vi "DAQ.vi"() -> ()   [LabVIEW 2018]
uses:
  55be89dd-8425-478b-abe4-e99fbfe30e24.vi
  <extravilib>/ChannelInstances/Messenger-bool/Write With Abort.vi
  <extravilib>/ChannelInstances/Messenger-bool/Read With Abort.vi
  <resource>/Channels/Messenger/Write With Abort.vi
  <resource>/Channels/Messenger/Read With Abort.vi
  <vilib>/ChannelSupport/Channel Message/Read ID.vi
  <extravilib>/ChannelInstances/Messenger-bool/Wrapper.lvclass
  C:/Program Files (x86)/National Instruments/LabVIEW 2018/vi.lib/ChannelSupport/Channel Message/Channel Message.lvclass
  <extravilib>/ChannelInstances/Messenger-bool/Instantiate.vi
  <resource>/Channels/Messenger/Endpoint.vi
  <extravilib>/ChannelInstances/Messenger-bool/Unwrap.vi
  <vilib>/Utility/inputDevices.llb/keyboardAcquire.vi
  <extravilib>/ChannelInstances/Messenger-bool/Wrap.vi
  PostgreSQL2LabVIEW/libpqlv/libpqlv.lvlib
  <vilib>/Utility/error.llb/DialogType.ctl
  <extravilib>/ChannelInstances/Messenger-bool.lvlib
panel:
  out "Chamber Temperature":dbl format="%#.1f °C"
  out "Chamber Pressure":dbl format="%#.1f psi"
  in  "CV-006\nAir Supply Valve":bool
  out "Pneumatic\nAir Pressure":dbl caption="Lox Tank Level" format="%#.1f psi"
  in  "CV-001\nFuel Vent Valve":bool
  out "Fuel Tank Pressure":dbl caption="Lox Tank Level" format="%#.1f psi"
  out "Thrust":dbl format="%#.0f N"
  out "Fuel Tank Level":dbl caption="Lox Tank Level" format="%#.1f kg"
  out "Fuel Tank Temperature":dbl format="%#.1f  °C"
  out "Lox Tank Level":dbl format="%#.1f  kg"
  out "LOX Tank Temperature":dbl format="%#.1f °C"
  in  "Start / Abort Button":bool
  out "data out":string
  out "Database Time":string
  out "Timer":string
  in  "stop":bool
  out "Fuel Feed Pressure":dbl format="%#.1f psi"
  out "LOX Feed Pressure":dbl format="%#.1f psi"
  out "Helium Pressure":dbl format="%#.0f psi"
  out "LOX Tank Pressure":dbl format="%#.1f psi"
  in  "CV-005\nLOX Fill Valve":bool
  in  "CV-003\nMain LOX Valve":bool
  in  "CV-002\nLOX Vent Valve":bool
  in  "CV-000\nHelium Valve":bool
  in  "CV-004\nMain Fuel Valve":bool
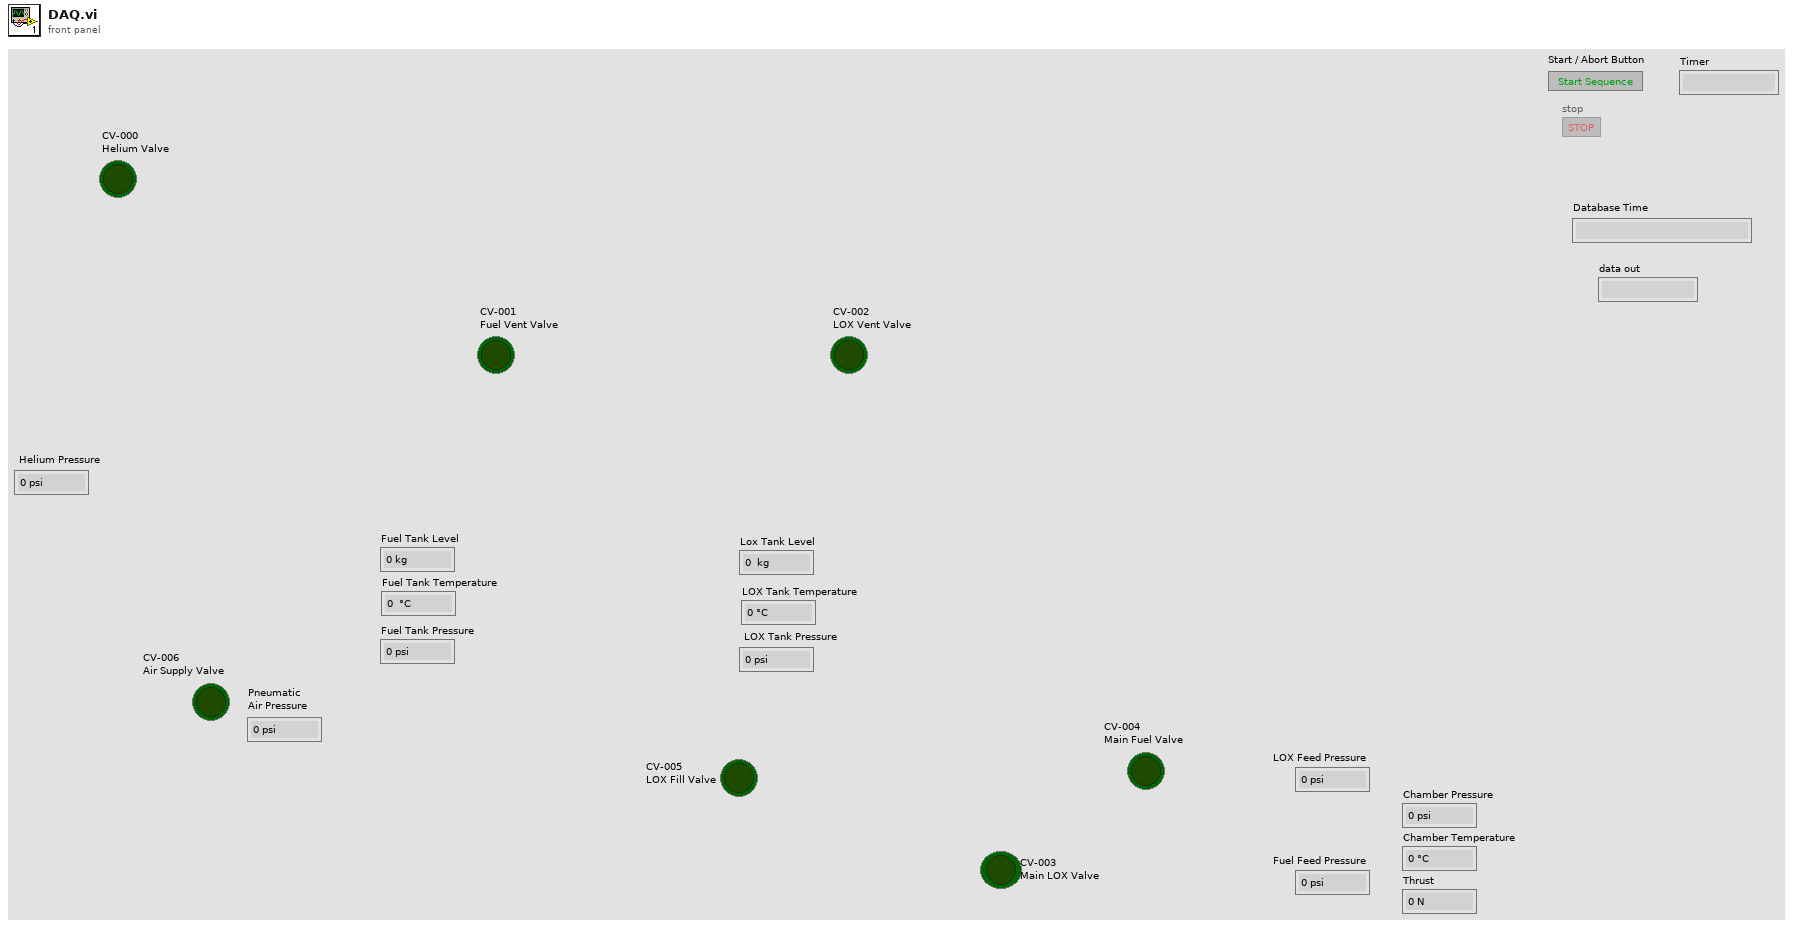
[diagram p1: front panel]
types:
  T1 = enum8{"Enabled", "Disabled", "Disabled and Grayed Out"}
  T2 = enum16{"0", "1", "2", "3", "4", "5", "6", "7", "8", "9", "A", "B", "C", "D", "E", "F", "G", "H", "I", "J", "K", "L", "M", "N", "O", "P", "Q", "R", "S", "T", "U", "V", "W", "X", "Y", "Z", "F1", "F2", "F3", "F4", "F5", "F6", "F7", "F8", "F9", "F10", "F11", "F12", "F13", "F14", "F15", "ADD", "BACK", "BACKSLASH", "CAPITAL", "COMMA", "DECIMAL", "DELETE", "DIVIDE", "DOWN", "END", "EQUALS", "ESCAPE", "GRAVE (`)", "HOME", "INSERT", "LBRACKET", "LCONTROL", "LEFT", "L ALT", "LSHIFT", "LWIN", "MINUS", "MULTIPLY", "NEXT", "NUMLOCK", "NUMPAD_0", "NUMPAD_1", "NUMPAD_2", "NUMPAD_3", "NUMPAD_4", "NUMPAD_5", "NUMPAD_6", "NUMPAD_7", "NUMPAD_8", "NUMPAD_9", "PAUSE", "PERIOD", "PRIOR (PG UP)", "RBRACKET", "RCONTROL", "RETURN", "RIGHT", "R ALT", "RSHIFT", "RWIN", "SCROLL", "SEMICOLON", "SLASH", "SPACE", "SUBTRACT", "TAB", "UP", "ENTER (num pad)", "' (quote)"}
  T3 = enum16{"0", "1", "2", "3", "4", "5", "6", "7", "8", "9", "A", "B", "C", "D", "E", "F", "G", "H", "I", "J", "K", "L", "M", "N", "O", "P", "Q", "R", "S", "T", "U", "V", "W", "X", "Y", "Z", "F1", "F2", "F3", "F4", "F5", "F6", "F7", "F8", "F9", "F10", "F11", "F12", "F13", "F14", "F15", "ADD", "BACK", "BACKSLASH", "CAPITAL", "COMMA", "DECIMAL", "DELETE", "DIVIDE", "DOWN", "END", "EQUALS", "ESCAPE", "GRAVE (`)", "HOME", "INSERT", "LBRACKET", "LCONTROL", "LEFT", "L ALT", "LSHIFT", "LWIN", "MINUS", "MULTIPLY", "NEXT", "NUMLOCK", "NUMPAD_0", "NUMPAD_1", "NUMPAD_2", "NUMPAD_3", "NUMPAD_4", "NUMPAD_5", "NUMPAD_6", "NUMPAD_7", "NUMPAD_8", "NUMPAD_9", "PAUSE", "PERIOD", "PRIOR (PG UP)", "RBRACKET", "RCONTROL", "RETURN", "RIGHT", "R ALT", "RSHIFT", "RWIN", "SCROLL", "SEMICOLON", "SLASH", "SPACE", "SUBTRACT", "TAB", "UP", "ENTER (num pad)", "' (quote)"}[]
  T4 = typedef "Messenger-bool.lvlib/))Channel.ctl" = refnum<queue>
  T5 = enum16{"Standard", "Buffered", "CRLF", "Immediate"}
  T6 = typedef "DialogType.ctl" = u16
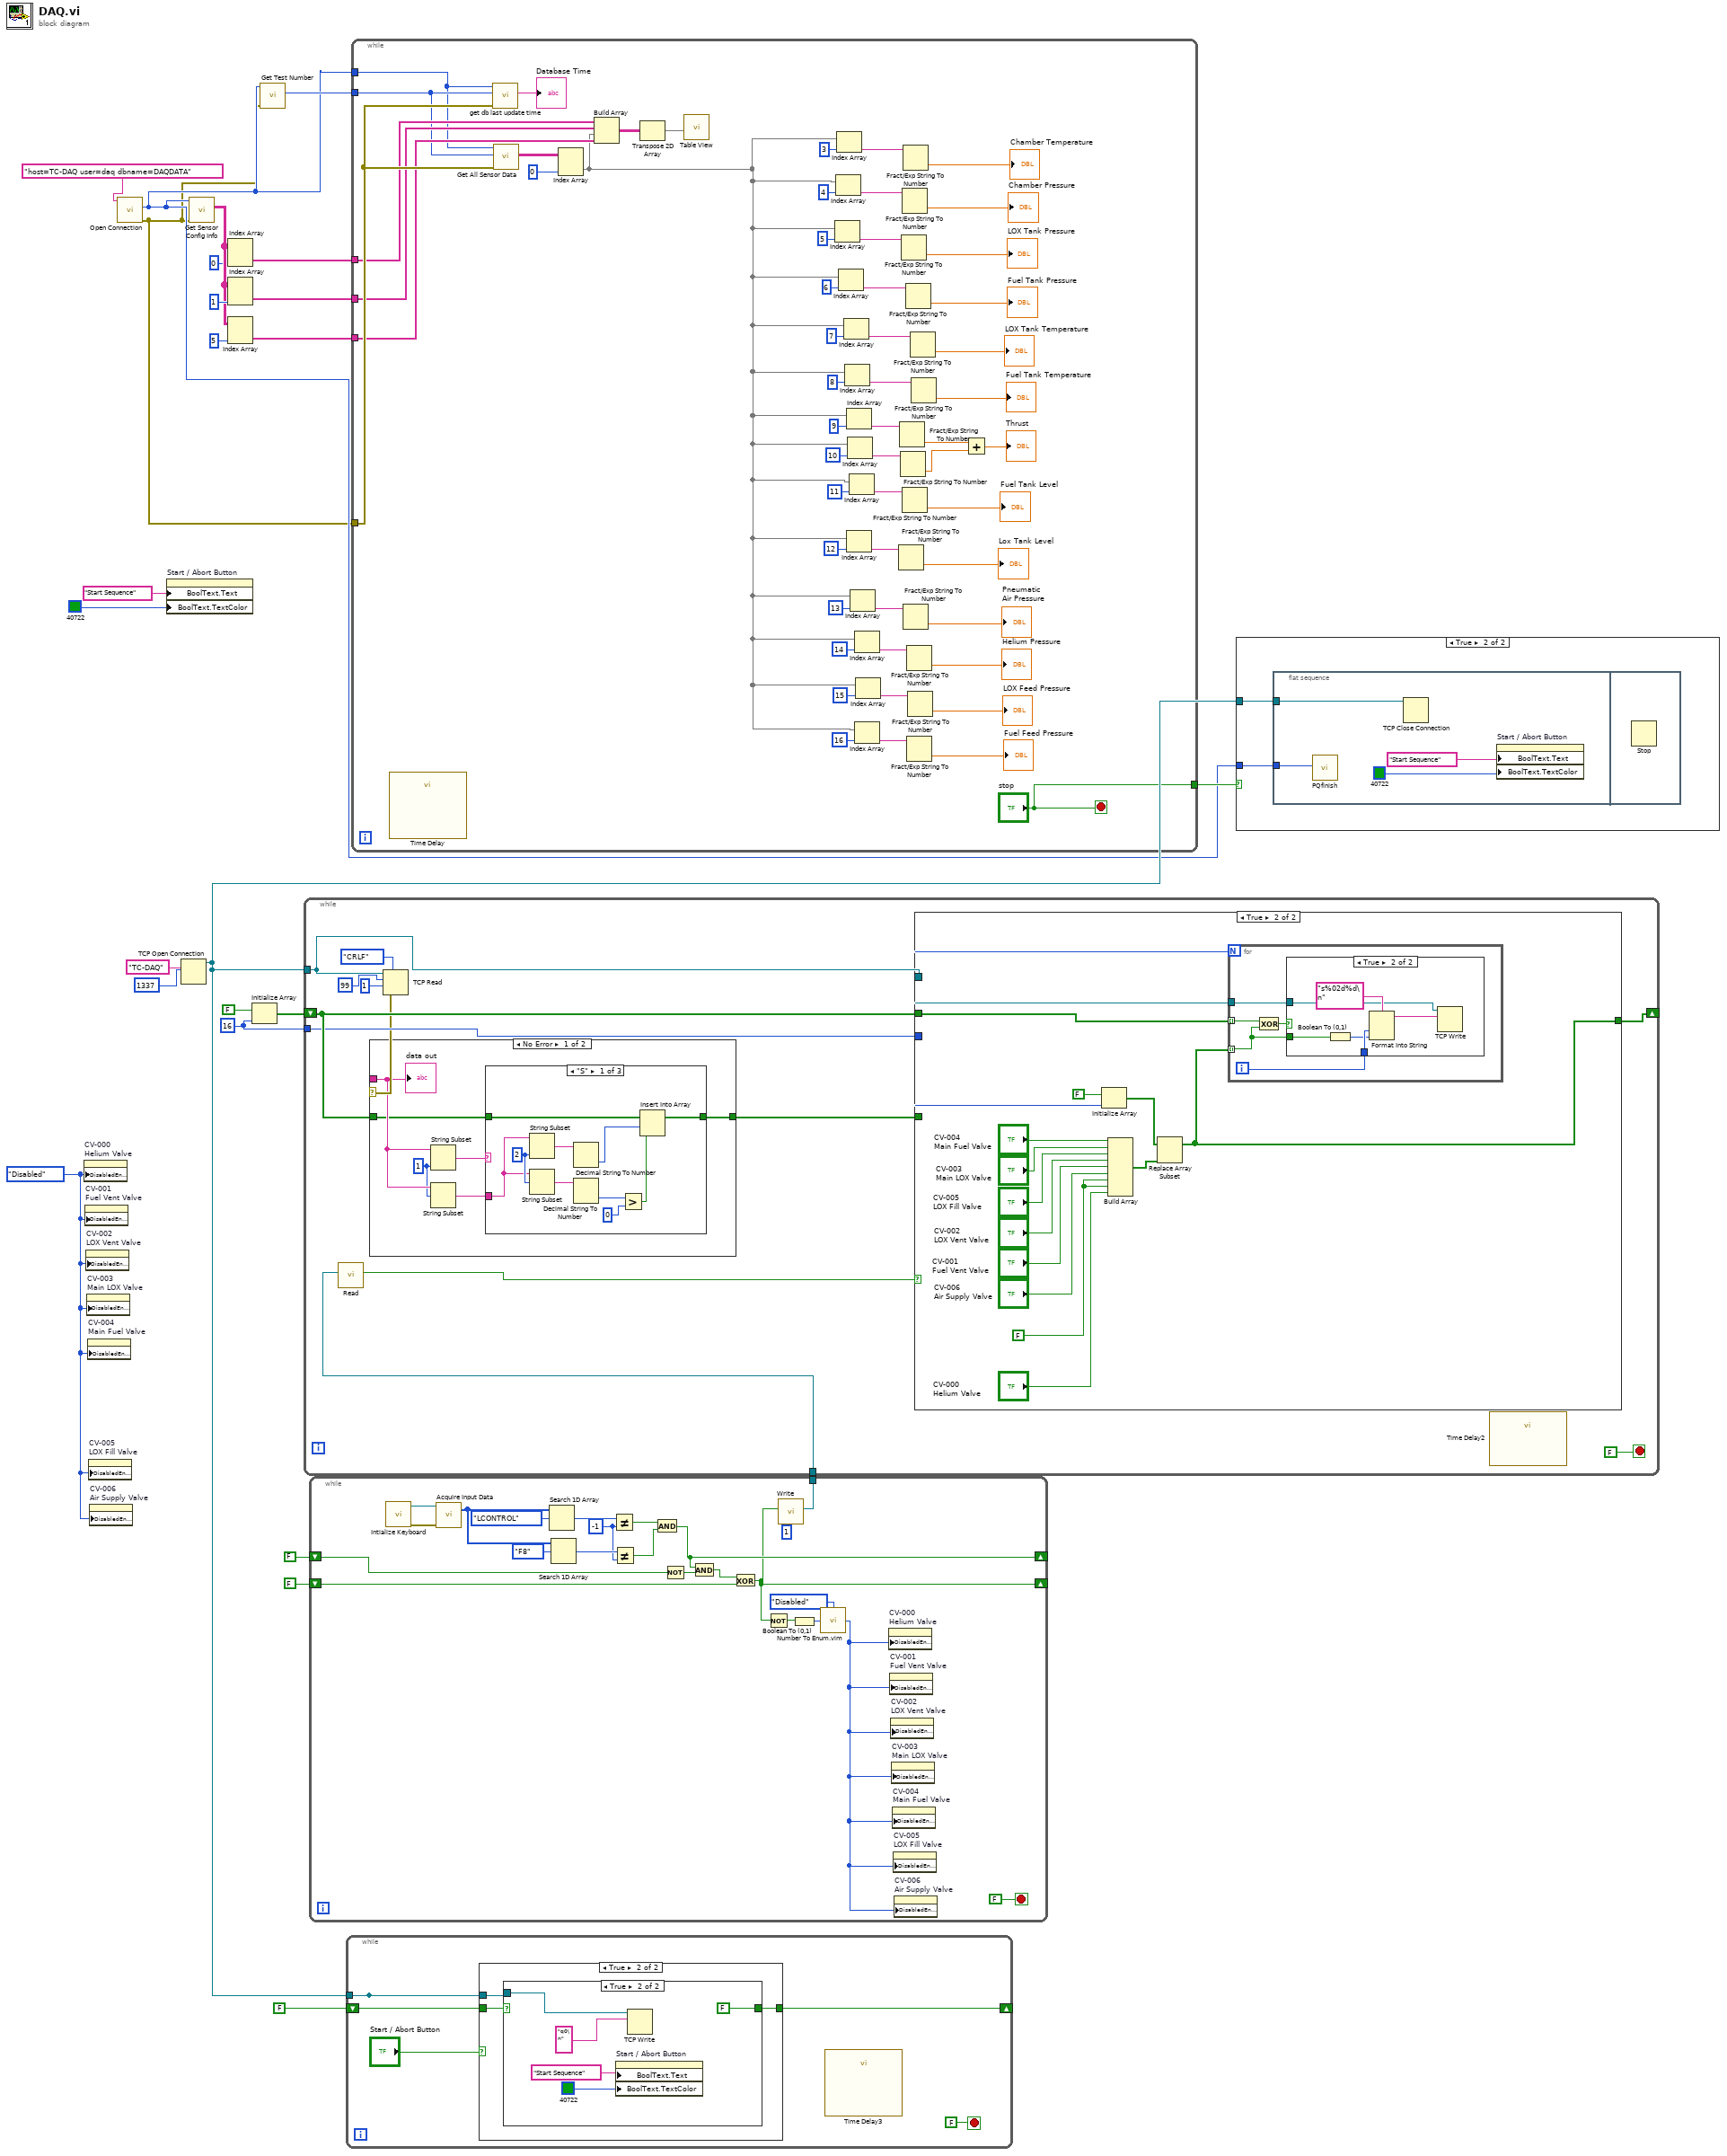
[diagram p0: block diagram]
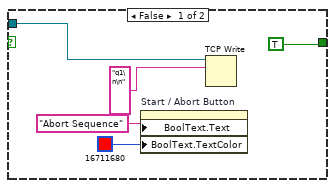
[diagram p3: hidden frame]
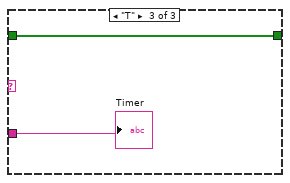
[diagram p5: hidden frame]
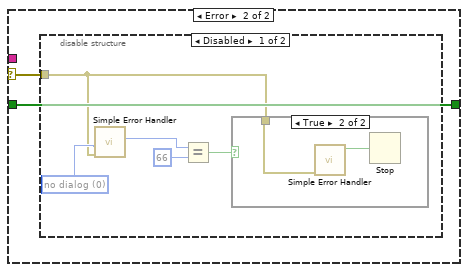
[diagram p6: hidden frame]
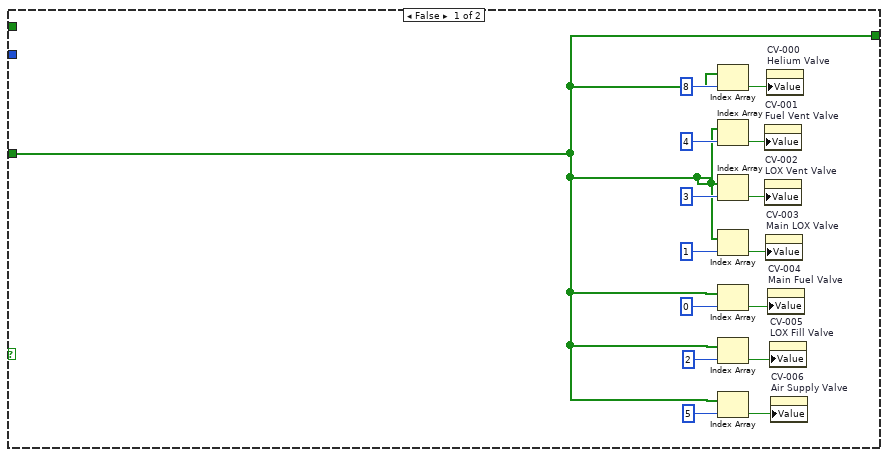
[diagram p9: hidden frame]
diagram:
  w7 = T1."Disabled" ("Disabled")
  w3 = 16 ("dimension size")
  n1 = property on="CV-000\nHelium Valve" class="Bool (strict)"("DisabledEnum"=w7) -> ()  [unwired: 2 in, 2 out]
  n2 = property on="CV-001\nFuel Vent Valve" class="Bool (strict)"("DisabledEnum"=w7) -> ()  [unwired: 2 in, 2 out]
  n3 = property on="CV-002\nLOX Vent Valve" class="Bool (strict)"("DisabledEnum"=w7) -> ()  [unwired: 2 in, 2 out]
  n4 = property on="CV-003\nMain LOX Valve" class="Bool (strict)"("DisabledEnum"=w7) -> ()  [unwired: 2 in, 2 out]
  n5 = property on="CV-004\nMain Fuel Valve" class="Bool (strict)"("DisabledEnum"=w7) -> ()  [unwired: 2 in, 2 out]
  n6 = property on="CV-005\nLOX Fill Valve" class="Bool (strict)"("DisabledEnum"=w7) -> ()  [unwired: 2 in, 2 out]
  n7 = property on="CV-006\nAir Supply Valve" class="Bool (strict)"("DisabledEnum"=w7) -> ()  [unwired: 2 in, 2 out]
  n8 = call "Open Connection.vi"("conninfo"="host=TC-DAQ user=daq dbname=DAQDATA") -> ("error out"=w1:errorcluster, "conn"=w2:u32)  [unwired: 8 in, 1 out]
  n9 = property on="Start / Abort Button" class="Bool"("BoolText.Text"="Start Sequence" ("Boolean Text.Text"), "BoolText.TextColor"=u32 40722) -> ()  [unwired: 2 in, 2 out]
  n10 = TCP Open Connection(address="TC-DAQ", remote port or service name=u16 1337) -> (connection ID=w17:refnum<k5>)  [unwired: 3 in, 1 out]
  n11 = call "Get Sensor Config Info.vi"("error in"=w1, "conn"=w2) -> ("Data"=w10:string[][])  [unwired: 7 in, 2 out]
  n12 = Index Array(array=w10, index (col)=0 ("disabled index (col)")) -> (element=w8:string[])  [unwired: 1 in]
  n13 = Index Array(array=w10, index (col)=1) -> (element=w13:string[])  [unwired: 1 in]
  n14 = Index Array(array=w10, index (col)=5 ("disabled index (col)")) -> (element=w11:string[])  [unwired: 1 in]
  n15 = Initialize Array(FALSE, w3) -> (w15:bool[])
  n16 = call "Get Test Number.vi"("error in"=w1, "conn"=w2) -> ("test_num"=w24:i32)  [unwired: 7 in, 2 out]
  n17 = while {
    shift-right: [w37] -> _
    shift-left: FALSE -> [w35]
    shift-right: [w31] -> _
    shift-left: FALSE -> [w33]
    tunnel: [w27] -> w4
    stop <- FALSE stop-if-true
    w40 = -1 ("y")
    n18 = call <vilib>:"Intialize Keyboard.vi"() -> ("error out"=w46:errorcluster, "device ID"=w48:refnum<k1>)  [unwired: 10 in]
    n19 = call-poly <vilib>:"Acquire Input Data.vi"("device ID"=w48, "error in (no error)"=w46) -> ("keys pressed"=w44:T3)  [unwired: 15 in, 2 out]
    n20 = Search 1D Array(1D array=w44, element=T2."LCONTROL") -> (index of element=w42:i32)  [unwired: 1 in]
    n21 = Search 1D Array(1D array=w44, element=T2."F8") -> (index of element=w41:i32)  [unwired: 1 in]
    n22 = Not Equal?(x=w42, y=w40) -> (x != y?=w39:bool)
    n23 = Not Equal?(x=w41, y=w40) -> (x != y?=w38:bool)
    n24 = And(x=w39, y=w38) -> (x .and. y?=w37:bool)
    n25 = Not(x=w35) -> (.not. x?=w36:bool)
    n26 = And(x=w37, y=w36) -> (x .and. y?=w34:bool)
    n27 = Exclusive Or(1:w33, 2:w34) -> (0:w31:bool)
    n28 = Not(x=w31) -> (.not. x?=w32:bool)
    n29 = call <extravilib>:"Write.vi"("size (unlimited)"=1, "element"=w31) -> ("channel"=w27:T4)  [unwired: 7 in, 2 out]
    n30 = Boolean To (0,1)(Boolean=w32) -> (0, 1=w30:i16)
    n31 = call "Number To Enum.vim"("number"=w30, "enum type"=T1."Disabled" ("Disabled")) -> ("number as enum"=w29:T1)
    n32 = property on="CV-000\nHelium Valve" class="Bool (strict)"("DisabledEnum"=w29) -> ()  [unwired: 2 in, 2 out]
    n33 = property on="CV-001\nFuel Vent Valve" class="Bool (strict)"("DisabledEnum"=w29) -> ()  [unwired: 2 in, 2 out]
    n34 = property on="CV-002\nLOX Vent Valve" class="Bool (strict)"("DisabledEnum"=w29) -> ()  [unwired: 2 in, 2 out]
    n35 = property on="CV-003\nMain LOX Valve" class="Bool (strict)"("DisabledEnum"=w29) -> ()  [unwired: 2 in, 2 out]
    n36 = property on="CV-004\nMain Fuel Valve" class="Bool (strict)"("DisabledEnum"=w29) -> ()  [unwired: 2 in, 2 out]
    n37 = property on="CV-005\nLOX Fill Valve" class="Bool (strict)"("DisabledEnum"=w29) -> ()  [unwired: 2 in, 2 out]
    n38 = property on="CV-006\nAir Supply Valve" class="Bool (strict)"("DisabledEnum"=w29) -> ()  [unwired: 2 in, 2 out]
  }
  n39 = while {
    tunnel: w17 -> [w61]
    shift-right: [w49] -> _
    shift-left: w15 -> [w60]
    tunnel: w4 -> [w58]
    tunnel: w3 -> [w56]
    stop <- FALSE stop-if-true
    n40 = call <extravilib>:"Read.vi"("channel"=w58) -> ("element"=w57:bool)  [unwired: 7 in, 3 out]
    n41 = TCP Read(connection ID=w61, bytes to read=99, 7:T5."CRLF" ("mode (standard)"), 9:1 ("timeout ms (25000)")) -> (data out=w54:string, error out=w55:errorcluster)  [unwired: 1 in, 1 out]
    n42 = case shown="No Error" w55 {
      selector: w55 -> [_ w81]
      tunnel: w54 -> [w66 _]
      tunnel: w60 -> [w63 w82]
      tunnel: [w62 w82] -> w51
      frame No Error {
        w65 = 1 ("length (rest)")
        n43 = String Subset(string=w66, length (rest)=w65) -> (substring=w67:string)  [unwired: 1 in]
        n44 = String Subset(string=w66, offset (0)=w65) -> (substring=w64:string)  [unwired: 1 in]
        n45 = case shown="\"S\"" w67 {
          tunnel: w64 -> [w68 _ w80]
          tunnel: w63 -> [w77 w78 w79]
          tunnel: [w69 w78 w79] -> w62
          frame "S" {
            w74 = 2 ("length (rest)")
            n46 = String Subset(string=w68, length (rest)=w74) -> (substring=w76:string)  [unwired: 1 in]
            n47 = String Subset(string=w68, offset (0)=w74) -> (substring=w73:string)  [unwired: 1 in]
            n48 = Decimal String To Number(string=w76) -> (number=w75:i32)  [unwired: 2 in, 1 out]
            n49 = Decimal String To Number(string=w73) -> (number=w72:i32)  [unwired: 2 in, 1 out]
            n50 = Greater?(x=w72, y=0) -> (0:w70:bool)
            n51 = Insert Into Array(array=w77, index=w75, new element=w70) -> (w69:bool[])
          }
          frame "False", Default {
          }
          frame "T" {
            "Timer" <- w80
          }
        }
        "data out" <- w66
      }
      frame Error {
        n52 = disable-structure shown="Disabled" {
          disable-tunnel: w81 -> [w83 _]
          frame Disabled {
            w85 = T6 0 items=["no dialog", "OK message", "continue or stop message", "OK message + warnings", "continue/stop + warnings"] ("type of dialog (OK msg:1)")
            n53 = call <vilib>:"Simple Error Handler.vi"("type of dialog (OK msg:1)"=w85, "error in (no error)"=w83) -> ("code out"=w84:i32)  [unwired: 3 in, 4 out]
            n54 = Equal?(x=w84, y=66) -> (x = y?=w86:bool)
            n55 = case shown="True" w86 {
              tunnel: w83 -> [_ w89]
              frame False {
              }
              frame True {
                n56 = call <vilib>:"Simple Error Handler.vi"("error in (no error)"=w89) -> ("error?"=w88:bool)  [unwired: 4 in, 4 out]
                n57 = Stop(stop? (T)=w88) -> ()
              }
            }
          }
          frame Enabled {
          }
        }
      }
    }
    n58 = case shown="True" w57 {
      tunnel: w61 -> [_ w113]
      tunnel: w60 -> [_ w114]
      tunnel: [w90 w115] -> w49
      tunnel: w56 -> [_ w116]
      tunnel: w51 -> [w90 _]
      frame False {
        n59 = Index Array(array=w90, index=8) -> (element=w97:bool)
        n60 = Index Array(array=w90, index=4) -> (element=w96:bool)
        n61 = Index Array(array=w90, index=3) -> (element=w98:bool)
        n62 = Index Array(array=w90, index=1) -> (element=w95:bool)
        n63 = Index Array(array=w90, index=0) -> (element=w94:bool)
        n64 = Index Array(array=w90, index=2) -> (element=w93:bool)
        n65 = Index Array(array=w90, index=5) -> (element=w91:bool)
        n66 = property on="CV-001\nFuel Vent Valve" class="Bool (strict)"("Value"=w96) -> ()  [unwired: 2 in, 2 out]
        n67 = property on="CV-002\nLOX Vent Valve" class="Bool (strict)"("Value"=w98) -> ()  [unwired: 2 in, 2 out]
        n68 = property on="CV-003\nMain LOX Valve" class="Bool (strict)"("Value"=w95) -> ()  [unwired: 2 in, 2 out]
        n69 = property on="CV-000\nHelium Valve" class="Bool (strict)"("Value"=w97) -> ()  [unwired: 2 in, 2 out]
        n70 = property on="CV-004\nMain Fuel Valve" class="Bool (strict)"("Value"=w94) -> ()  [unwired: 2 in, 2 out]
        n71 = property on="CV-005\nLOX Fill Valve" class="Bool (strict)"("Value"=w93) -> ()  [unwired: 2 in, 2 out]
        n72 = property on="CV-006\nAir Supply Valve" class="Bool (strict)"("Value"=w91) -> ()  [unwired: 2 in, 2 out]
      }
      frame True {
        w106 = FALSE
        n73 = Initialize Array(FALSE, w116) -> (w118:bool[])
        n74 = Build Array("CV-004\nMain Fuel Valve", "CV-003\nMain LOX Valve", "CV-005\nLOX Fill Valve", "CV-002\nLOX Vent Valve", "CV-001\nFuel Vent Valve", "CV-006\nAir Supply Valve", w106, w106, "CV-000\nHelium Valve") -> (w117:bool[])
        n75 = Replace Array Subset(array=w118, new element=w117) -> (w115:bool[])  [unwired: 1 in]
        n76 = for {
          N: w116 -> [_]
          tunnel: w115 -> [w120] mode=indexing
          tunnel: w114 -> [w124] mode=indexing
          tunnel: w113 -> [w122]
          i -> [w121]
          n77 = Exclusive Or(1:w120, 2:w124) -> (0:w123:bool)
          n78 = case shown="True" w123 {
            tunnel: w122 -> [_ w126]
            tunnel: w121 -> [_ w129]
            tunnel: w120 -> [_ w128]
            frame False {
            }
            frame True {
              n79 = Boolean To (0,1)(Boolean=w128) -> (0, 1=w125:i16)
              n80 = Format Into String(format string="s%02d%d\n", w129, w125) -> (resulting string=w127:string)  [unwired: 2 in, 1 out]
              n81 = TCP Write(connection ID=w126, data in=w127) -> ()  [unwired: 2 in, 3 out]
            }
          }
        }
      }
    }
    n82 = call "Time Delay2"() -> ()  [unwired: 11 in, 1 out]
  }
  n83 = while {
    tunnel: w17 -> [w132]
    shift-right: [w135] -> _
    shift-left: FALSE -> [w134]
    tunnel: [w132] -> _
    stop <- FALSE stop-if-true
    n84 = case shown="True" "Start / Abort Button" {
      tunnel: w132 -> [_ w139]
      tunnel: [w136 w138] -> w135
      tunnel: w134 -> [w136 w137]
      frame False {
      }
      frame True {
        n85 = case shown="True" w137 {
          tunnel: w139 -> [w142 w148]
          tunnel: [TRUE FALSE] -> w138
          frame False {
            n86 = property on="Start / Abort Button" class="Bool"("BoolText.Text"="Abort Sequence" ("Boolean Text.Text"), "BoolText.TextColor"=u32 16711680) -> ()  [unwired: 2 in, 2 out]
            n87 = TCP Write(connection ID=w142, data in="q1\n\n") -> ()  [unwired: 2 in, 3 out]
          }
          frame True {
            n88 = property on="Start / Abort Button" class="Bool"("BoolText.Text"="Start Sequence" ("Boolean Text.Text"), "BoolText.TextColor"=u32 40722) -> ()  [unwired: 2 in, 2 out]
            n89 = TCP Write(connection ID=w148, data in="q0\n") -> ()  [unwired: 2 in, 3 out]
          }
        }
      }
    }
    n90 = call "Time Delay3"() -> ()  [unwired: 11 in, 1 out]
  }
  n91 = while {
    tunnel: w24 -> [w177]
    tunnel: w2 -> [w176]
    tunnel: w1 -> [w203]
    tunnel: ["stop"] -> w18
    tunnel: w13 -> [w200]
    tunnel: w11 -> [w199]
    tunnel: w8 -> [w195]
    stop <- "stop" stop-if-true
    n92 = call "Time Delay"() -> ()  [unwired: 11 in, 1 out]
    n93 = call "get db last update time.vi"("error in"=w203, "test_num"=w177, "conn"=w176) -> ("field_value"=→"Database Time":string)  [unwired: 7 in, 1 out]
    n94 = call "Get All Sensor Data.vi"("error in"=w203, "test_num"=w177, "conn"=w176) -> ("Data"=w202:string[][])  [unwired: 6 in, 2 out]
    n95 = Index Array(array=w202, index (col)=0 ("disabled index (col)")) -> (element=w150:string[])  [unwired: 1 in]
    n96 = Build Array(w195, w200, w150, w199) -> (w198:string[][])
    n97 = Transpose 2D Array(2D array=w198) -> (transposed array=w197:string[][])
    n98 = call "Table View.vi"("Table"=w197) -> ()  [unwired: 11 in]
    n99 = Index Array(array=w150, index=5) -> (element=w187:string)
    n100 = Index Array(array=w150, index=4) -> (element=w155:string)
    n101 = Index Array(array=w150, index=3) -> (element=w152:string)
    n102 = Index Array(array=w150, index=6) -> (element=w178:string)
    n103 = Index Array(array=w150, index=7) -> (element=w182:string)
    n104 = Index Array(array=w150, index=8) -> (element=w184:string)
    n105 = Index Array(array=w150, index=9) -> (element=w194:string)
    n106 = Index Array(array=w150, index=12) -> (element=w164:string)
    n107 = Index Array(array=w150, index=10) -> (element=w193:string)
    n108 = Index Array(array=w150, index=11) -> (element=w166:string)
    n109 = Index Array(array=w150, index=13) -> (element=w159:string)
    n110 = Index Array(array=w150, index=14) -> (element=w169:string)
    n111 = Index Array(array=w150, index=16) -> (element=w175:string)
    n112 = Index Array(array=w150, index=15) -> (element=w172:string)
    n113 = Fract/Exp String To Number(string=w164) -> (number=→"Lox Tank Level":dbl)  [unwired: 3 in, 1 out]
    n114 = Fract/Exp String To Number(string=w194) -> (number=w191:dbl)  [unwired: 3 in, 1 out]
    n115 = Fract/Exp String To Number(string=w193) -> (number=w190:dbl)  [unwired: 3 in, 1 out]
    n116 = Fract/Exp String To Number(string=w187) -> (number=→"LOX Tank Pressure":dbl)  [unwired: 3 in, 1 out]
    n117 = Fract/Exp String To Number(string=w155) -> (number=→"Chamber Pressure":dbl)  [unwired: 3 in, 1 out]
    n118 = Fract/Exp String To Number(string=w166) -> (number=→"Fuel Tank Level":dbl)  [unwired: 3 in, 1 out]
    n119 = Fract/Exp String To Number(string=w152) -> (number=→"Chamber Temperature":dbl)  [unwired: 3 in, 1 out]
    n120 = Fract/Exp String To Number(string=w159) -> (number=→"Pneumatic\nAir Pressure":dbl)  [unwired: 3 in, 1 out]
    n121 = Fract/Exp String To Number(string=w178) -> (number=→"Fuel Tank Pressure":dbl)  [unwired: 3 in, 1 out]
    n122 = Fract/Exp String To Number(string=w169) -> (number=→"Helium Pressure":dbl)  [unwired: 3 in, 1 out]
    n123 = Fract/Exp String To Number(string=w175) -> (number=→"Fuel Feed Pressure":dbl)  [unwired: 3 in, 1 out]
    n124 = Fract/Exp String To Number(string=w172) -> (number=→"LOX Feed Pressure":dbl)  [unwired: 3 in, 1 out]
    n125 = Fract/Exp String To Number(string=w182) -> (number=→"LOX Tank Temperature":dbl)  [unwired: 3 in, 1 out]
    n126 = Fract/Exp String To Number(string=w184) -> (number=→"Fuel Tank Temperature":dbl)  [unwired: 3 in, 1 out]
    n127 = Add(x=w191, y=w190) -> (x+y=→"Thrust":dbl)
  }
  n128 = case shown="True" w18 {
    tunnel: w17 -> [_ w207]
    tunnel: w2 -> [_ w206]
    frame False {
    }
    frame True {
      n129 = flat-sequence {
        tunnel: w207 -> [w209]
        tunnel: w206 -> [w208]
        frame #0 {
          n130 = call "PQfinish.vi"("conn"=w208) -> ()  [unwired: 10 in, 1 out]
          n131 = TCP Close Connection(connection ID=w209) -> ()  [unwired: 2 in, 2 out]
          n132 = property on="Start / Abort Button" class="Bool"("BoolText.Text"="Start Sequence" ("Boolean Text.Text"), "BoolText.TextColor"=u32 40722) -> ()  [unwired: 2 in, 2 out]
        }
        frame #1 {
          n133 = Stop() -> ()  [unwired: 1 in]
        }
      }
    }
  }
